vi "Test_ClearValues_EmptyTable.vi"(8 "error in (no error)":errorcluster, 11 "TestCase in":refnum<class "TestCurrentValueTable.lvclass">) -> (0 "error out":errorcluster, 3 "TestCase out":refnum<class "TestCurrentValueTable.lvclass">)   [LabVIEW 2015, in "CurrentValueTable.lvlib" / "TestCurrentValueTable.lvclass"]
uses:
  TestCurrentValueTable.lvclass
  <vilib>/addons/_JKI Toolkits/VI Tester/TestCase.llb/TestCase.lvclass
  CurrentValueTable.lvclass
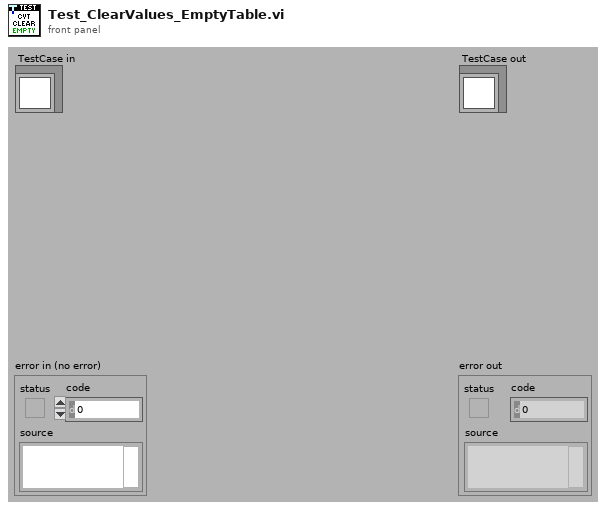
[diagram p1: front panel]
types:
  T1 = typedef "CurrentValueTable.lvlib/CurrentValueTable.lvclass/CurrentValueTable Reference.ctl" = refnum<data-value>
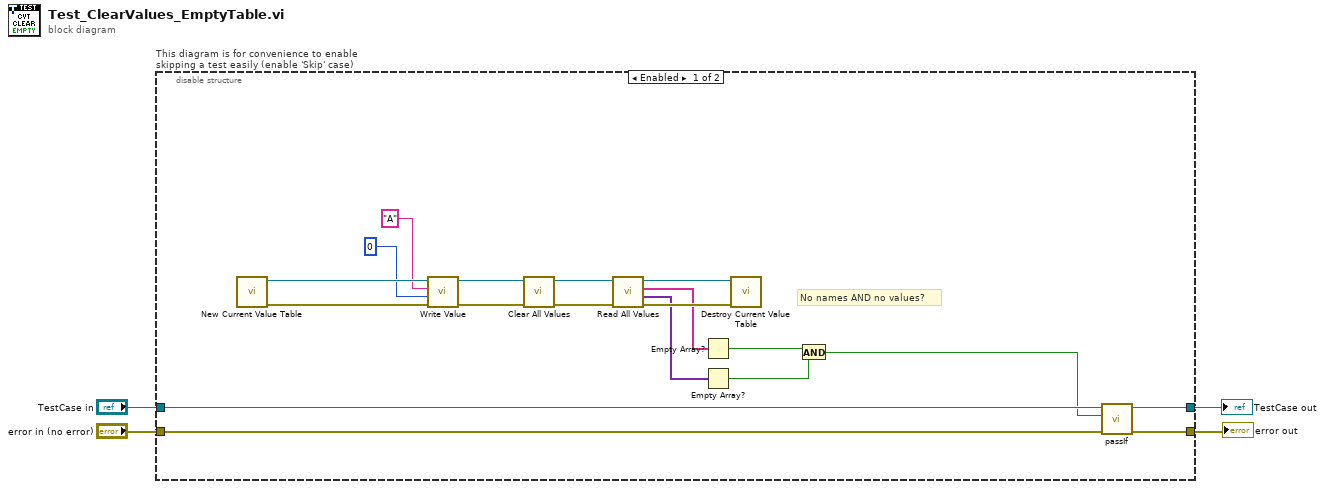
[diagram p0: block diagram]
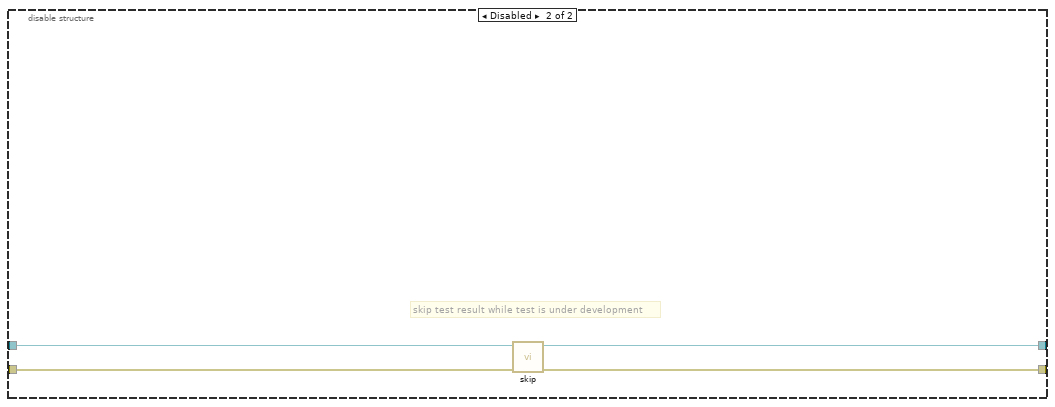
[diagram p2: hidden frame]
diagram:
  n1 = disable-structure "This diagram is for convenience to enable skipping a test easily (enable 'Skip' case)" shown="Enabled" {
    disable-tunnel: "TestCase in" -> [w23 w27]
    disable-tunnel: [w22 w25] -> w1
    disable-tunnel: [w21 w26] -> w3
    disable-tunnel: "error in (no error)" -> [w20 w24]
    frame Enabled {
      # "No names AND no values?"
      n2 = call "New Current Value Table.vi"() -> ("error out"=w15:errorcluster, "Current Value Table"=w19:T1)  [unwired: 10 in]
      n3 = call "Write Value.vi"("error in (no error)"=w15, "Value"=0, "Data Name (Use Value Name)"="A", "Current Value Table"=w19) -> ("error out"=w12:errorcluster, "Current Value Table"=w18:T1)  [unwired: 6 in]
      n4 = call "Clear All Values.vi"("error in (no error)"=w12, "Current Value Table"=w18) -> ("error out"=w11:errorcluster, "Current Value Table"=w14:T1)  [unwired: 8 in]
      n5 = call "Read All Values.vi"("error in (no error)"=w11, "Current Value Table"=w14) -> ("error out"=w10:errorcluster, "Values"=w9:variant[], "Names"=w8:string[], "Current Value Table"=w13:T1)  [unwired: 6 in]
      n6 = Empty Array?(array=w8) -> (empty?=w7:bool)
      n7 = Empty Array?(array=w9) -> (empty?=w6:bool)
      n8 = call "Destroy Current Value Table.vi"("error in (no error)"=w10, "Current Value Table"=w13) -> ()  [unwired: 9 in, 1 out]
      n9 = And(x=w7, y=w6) -> (x .and. y?=w5:bool)
      n10 = call-dynamic "passIf.vi"("error in (no error)"=w20, "pass"=w5, "TestCase in"=w23) -> ("error out"=w21:errorcluster, "TestCase out"=w22:refnum<class "TestCurrentValueTable.lvclass">)  [unwired: 7 in]
    }
    frame Disabled {
      # "skip test result while test is under development"
      n11 = call <vilib>:"skip.vi"("error in (no error)"=w24, "TestCase in"=w27) -> ("error out"=w26:errorcluster, "TestCase out"=w25:refnum<class "TestCurrentValueTable.lvclass">)  [unwired: 8 in]
    }
  }
  "error out" <- w3
  "TestCase out" <- w1
